vi "Init Msg Input.vi"(6 "Teller":T1 {"Time" format="%<%x %.3X>T"}) -> (2 "Msg Input":refnum<class "Msg Input.lvclass">)   [LabVIEW 2020, in "jettl.lvlib" / "Stop jettl Msg.lvlib" / "Stop Msg Input.lvlib"]
uses:
  Stop Msg Input.lvlib
  Msg Input/Msg Input.lvclass
  Stop Msg Input/Stop Msg Input.lvclass
  C:/git/jettl/src/jettl/jettl/Stop jettl Msg/Stop Msg Input/Stop Msg Input/Stop Msg Input.lvclass
  C:/git/jettl/src/jettl/jettl/Msg Input/Msg Input.lvclass
  Relation.ctl
  jettl.lvlib
  Teller Metadata/Teller Metadata.lvclass
  Teller.ctl
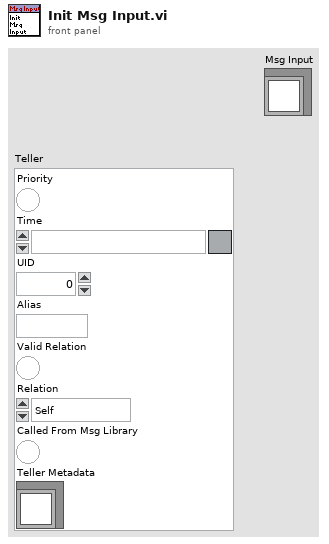
[diagram p1: front panel]
types:
  T1 = typedef "jettl.lvlib/Teller.ctl" = cluster{"Priority":bool, "Time":timestamp, "UID":i32, "Alias":string, "Valid Relation":bool, "Relation":T2, "Called From Msg Library":bool, "Teller Metadata":refnum<class "Teller Metadata.lvclass">}
  T2 = typedef "jettl.lvlib/Relation.ctl" = enum16{"Self", "Parent", "Child"}
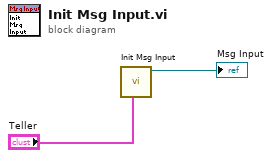
[diagram p0: block diagram]
diagram:
  n1 = call "Init Msg Input.vi"("Teller"="Teller") -> ("Stop Msg Input out"=→"Msg Input":refnum<class "Stop Msg Input.lvclass">)  [unwired: 10 in]
